vi "Set Ending Tangent.vi"(10 "waypts":cluster{"x":sgl, "y":sgl}[](array[cluster]), 11 "ending orientation":sgl=nan) -> (3 "ending tangent":cluster{sgl, sgl})   [LabVIEW 2025]
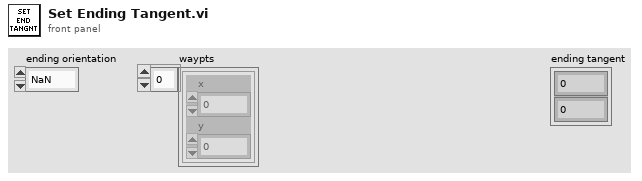
[diagram p1: front panel]
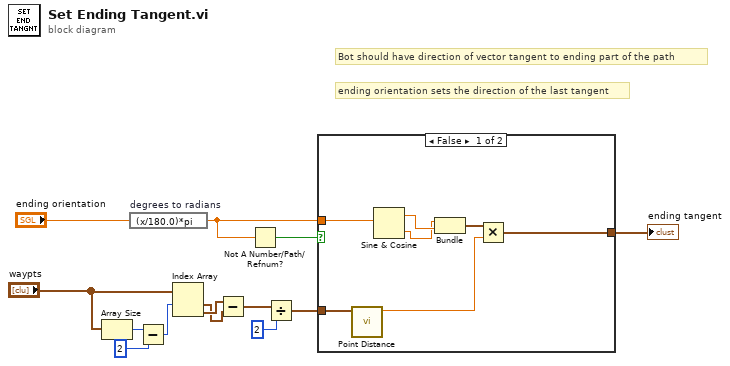
[diagram p0: block diagram]
diagram:
  # "Bot should have direction of vector tangent to ending part of the path"
  # "ending orientation sets the direction of the last tangent"
  n1 = Array Size(array="waypts") -> (size(s)=w12:i32)
  n2 = expression code="(x/180.0)*pi" "degrees to radians"("ending orientation") -> (w2:sgl)
  n3 = Subtract(x=w12, y=2) -> (x-y=w10:i32)
  n4 = Index Array(array="waypts", index #1=w10) -> (element #1=w8:cluster{"x":sgl, "y":sgl}, element #2=w9:cluster{"x":sgl, "y":sgl})  [unwired: 1 in]
  n5 = Subtract(x=w9, y=w8) -> (x-y=w5:cluster{"x":sgl, "y":sgl})
  n6 = Not A Number/Path/Refnum?(number/path/refnum=w2) -> (NaN/Path/Refnum?=w13:bool)
  n7 = Divide(x=w5, y=2) -> (x/y=w4:cluster{"x":sgl, "y":sgl})
  n8 = case shown="False" w13 {
    tunnel: w2 -> [w20 _]
    tunnel: [w16 w21] -> w7
    tunnel: w4 -> [w18 w21]
    frame False {
      n9 = call "Point Distance.vi"("point a"=w18) -> ("dist"=w17:sgl)  [unwired: 10 in]
      n10 = Sine & Cosine(0:w20) -> (1:w15:sgl, 2:w14:sgl)
      n11 = Bundle(w14, w15) -> (w19:cluster{sgl, sgl})  [unwired: 1 in]
      n12 = Multiply(x=w19, y=w17) -> (x*y=w16:cluster{sgl, sgl})
    }
    frame True {
    }
  }
  "ending tangent" <- w7
